vi "Test Rotate.vi"(8 "error in (no error)":errorcluster) -> (0 "error out":errorcluster)   [LabVIEW 2019]
uses:
  lvsrc/Instrument Types/Cryostat/Instrument.Cryostat.lvclass
  <vilib>/addons/_JKI Toolkits/Caraya/classes/Assert/Assert Error.vi
  <vilib>/addons/_JKI Toolkits/Caraya/classes/Assert/Assert Almost Equal_Float.vi
  <vilib>/addons/_JKI Toolkits/Caraya/classes/Assert/Assert.lvclass
  <vilib>/addons/_JKI Toolkits/Caraya/classes/Test/Test.lvclass
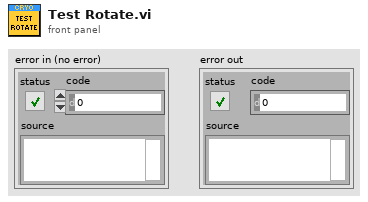
[diagram p1: front panel]
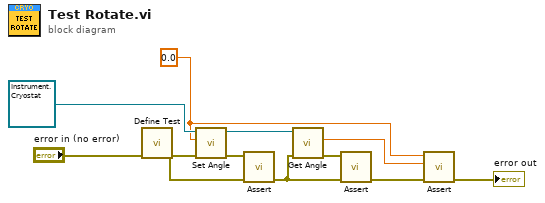
[diagram p0: block diagram]
diagram:
  w4 = 0.0 ("Angle (°)")
  n1 = call <vilib>:"Define Test.vi"("error in (no error)"="error in (no error)") -> ("error out"=w2:errorcluster)  [unwired: 10 in]
  n2 = call-dynamic "Set Angle.vi"("error in (no error)"=w2, "Angle (°)"=w4, "Instrument.Cryostat in"=refnum<class "Instrument.Cryostat.lvclass"> refnum) -> ("error out"=w11:errorcluster, "Instrument.Cryostat out"=w9:refnum<class "Instrument.Cryostat.lvclass">)  [unwired: 7 in]
  n3 = call-poly <vilib>:"Assert.vi"("error in (no error)"=w2, "Error?"=w11) -> ("error out"=w1:errorcluster)  [unwired: 9 in]
  n4 = call-dynamic "Get Angle.vi"("error in (no error)"=w1, "Instrument.Cryostat in"=w9) -> ("error out"=w7:errorcluster, "Angle (°)"=w6:dbl)  [unwired: 6 in, 2 out]
  n5 = call-poly <vilib>:"Assert.vi"("error in (no error)"=w1, "Error?"=w7) -> ("error out"=w5:errorcluster)  [unwired: 9 in]
  n6 = call-poly <vilib>:"Assert.vi"("error in (no error)"=w5, "Y"=w6, "X"=w4) -> ("error out"=→"error out":errorcluster)  [unwired: 8 in]
